vi "Read Index.vi"(8 "error in (no error)":errorcluster, 11 "Update CRD Housekeeping MSG in":refnum<class "Update CRD Housekeeping MSG.lvclass">) -> (0 "error out":errorcluster, 2 "Index":i32, 3 "Update CRD Housekeeping MSG out":refnum<class "Update CRD Housekeeping MSG.lvclass">)   [LabVIEW 2014, in "Update CRD Housekeeping MSG.lvclass"]
uses:
  Update CRD Housekeeping MSG.lvclass
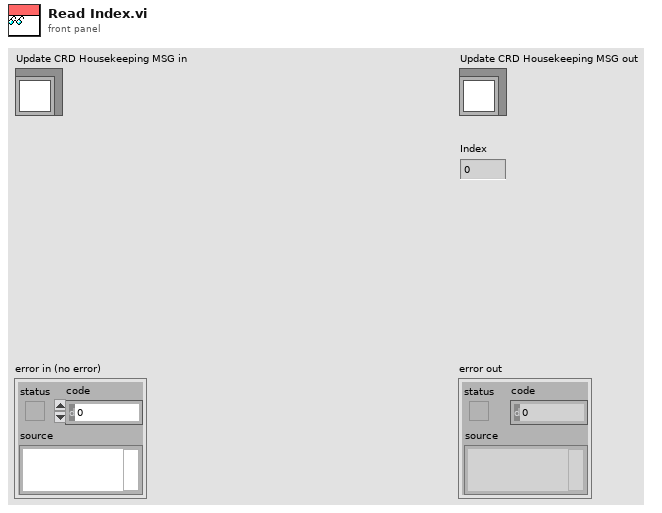
[diagram p1: front panel]
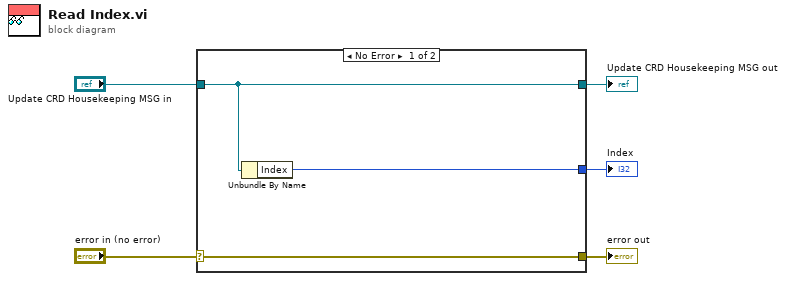
[diagram p0: block diagram]
diagram:
  n1 = case shown="No Error" "error in (no error)" {
    selector: "error in (no error)" -> [w8 w9]
    tunnel: [w8 w9] -> w4
    tunnel: [w7 w10] -> w2
    tunnel: "Update CRD Housekeeping MSG in" -> [w7 w10]
    tunnel: [w6 _] -> w1
    frame No Error {
      n2 = Unbundle By Name(w7) -> ("Index"=w6:i32)
    }
    frame Error {
    }
  }
  "error out" <- w4
  "Update CRD Housekeeping MSG out" <- w2
  "Index" <- w1
